vi "Global_CMD_ACT_Data In.vi"() -> ()   [LabVIEW 2023, in "SwerveDrive_ACT_ts.lvlib"]
uses:
  startup.rtexe/SwerveDrive_ACT_ts.lvlib
  Cluster_CMD_ACT_Data.ctl
  support/ENUM_CMD_Mode Select.ctl
  startup.rtexe/Cluster_CMD_Direction Data.ctl
  startup.rtexe/Cluster_Module Velocity-Direction-Rotations.ctl
  startup.rtexe/Level_Velocity plus-minus 1.ctl
  startup.rtexe/Dial_Compase heading unit circle CCW positive.ctl
  startup.rtexe/Cluster_X-Y.ctl
panel:
  in  "CMD_ACT_SwerveDrive_Data":T1 {"Auto Angle" scale format="%.3f"; "Direction"."Rotate(Yaw) CCW 1 CW -1" scale=1.0..-1.0; "Direction"."Traverse"."Angle" scale format="%.3f"; "Direction"."Traverse"."Velocity" scale=-1.0..1.0 scale format="%.1f"}
  # "The Names of the Data items in the Global Variable MUST describe who the Single Writer is\nFor Command Globals the Commander(CMD) represents Teleop or Autonomous or other command loop.\nThe naming convention for a Command Actuator Global is:   \n\nCMD_ACT_SubSystem_Data Name\n\nExample:\nCMD_ACT_Drive_Data\nCMD_ACT_Hopper_Eject Ball"
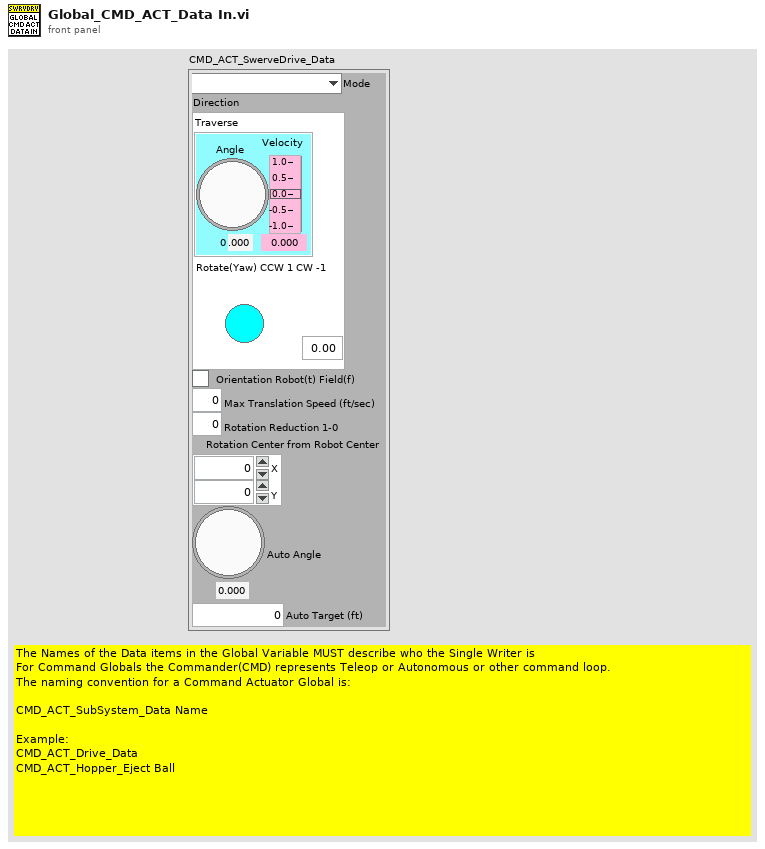
[diagram p1: front panel]
types:
  T1 = typedef "SwerveDrive_ACT_ts.lvlib/Cluster_CMD_ACT_Data.ctl" = cluster{"Mode":T2, "Direction":T3, "Orientation Robot(t) Field(f)":bool, "Max Translation Speed (ft/sec)":dbl, "Rotation Reduction 1-0":dbl, "Rotation Center from Robot Center":T7, "Auto Angle":T6, "Auto Target (ft)":dbl}
  T2 = typedef "ENUM_CMD_Mode Select.ctl" = enum16{"Stop", "Translate Cmd Rotate Cmd", "Translate Cmd Rotate Auto"}
  T3 = typedef "Cluster_CMD_Direction Data.ctl" = cluster{"Traverse":T4, "Rotate(Yaw) CCW 1 CW -1":dbl}
  T4 = typedef "Cluster_Module Velocity-Direction-Rotations.ctl" = cluster{"Velocity":T5, "Angle":T6, "Rotations Count":dbl}
  T5 = typedef "Level_Velocity plus-minus 1.ctl" = dbl
  T6 = typedef "Dial_Compase heading unit circle CCW positive.ctl" = dbl
  T7 = typedef "Cluster_X-Y.ctl" = cluster{"X":dbl, "Y":dbl}
diagram:
